vi "CMRR&PSRR.vi"(11 "数组":dbl[](array[numeric])) -> (2 "PSRR":dbl=122.60591675460435, 3 "KCMRR":dbl=118.45179628787717)   [LabVIEW 2019]
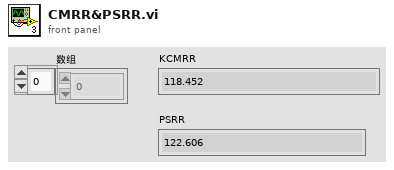
[diagram p1: front panel]
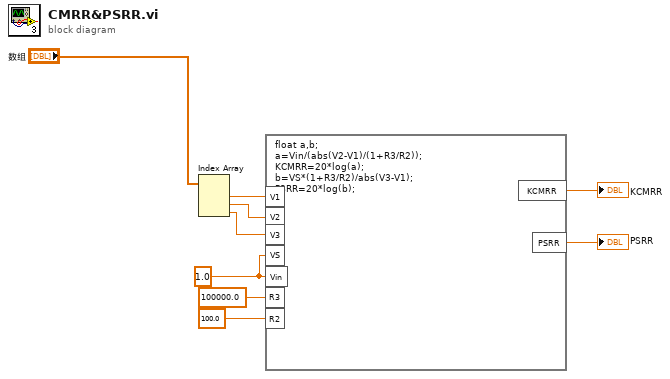
[diagram p0: block diagram]
diagram:
  w7 = 1.0 ("输入变量")
  n1 = Index Array(array="数组") -> (element #1=w1:dbl, element #2=w2:dbl, element #3=w6:dbl)  [unwired: 3 in]
  n2 = formula code="float a,b;\na=Vin/(abs(V2-V1)/(1+R3/R2));\nKCMRR=20*log(a);\nb=VS*(1+R3/R2)/abs(V3-V1);\nPSRR=20*log(b);"("V1"=w1, "V2"=w2, "R3"=100000.0 ("输入变量"), "R2"=100.0 ("输入变量"), "Vin"=w7, "VS"=w7, "V3"=w6) -> ("KCMRR"=→"KCMRR":dbl, "PSRR"=→"PSRR":dbl)
